vi "BT3562_CMD.vi"(8 "errin":errorcluster caption="entrée d'erreur (pas d'erreur)") -> (0 "errout":errorcluster caption="sortie d'erreur", 3 "Conti (mOhms)":dbl format="%#_10f")   [LabVIEW 2020]
uses:
  <vilib>/Instr/_visa.llb/VISA Find Search Mode.ctl
  <instrlib>/HIOKI BT356X Series/HIOKI BT356X Series.lvlib
panel:
  in  "errin":errorcluster caption="entrée d'erreur (pas d'erreur)"
  in  "visa in":refnum<visa-resource-name>
  out "Conti (Ohms)":dbl format="%#_10f"
  out "VISA OUT":string
  out "DATA OUT":string
  # "DATA OUT"
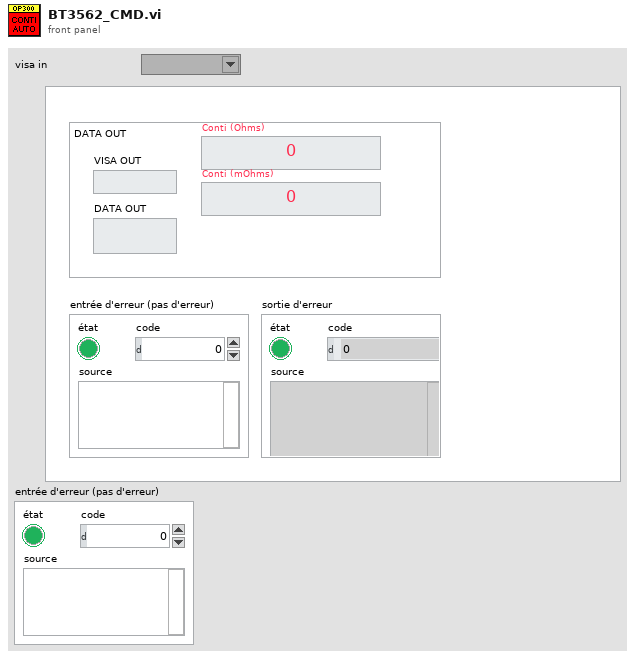
[diagram p1: front panel]
types:
  T1 = typedef "VISA Find Search Mode.ctl" = u32
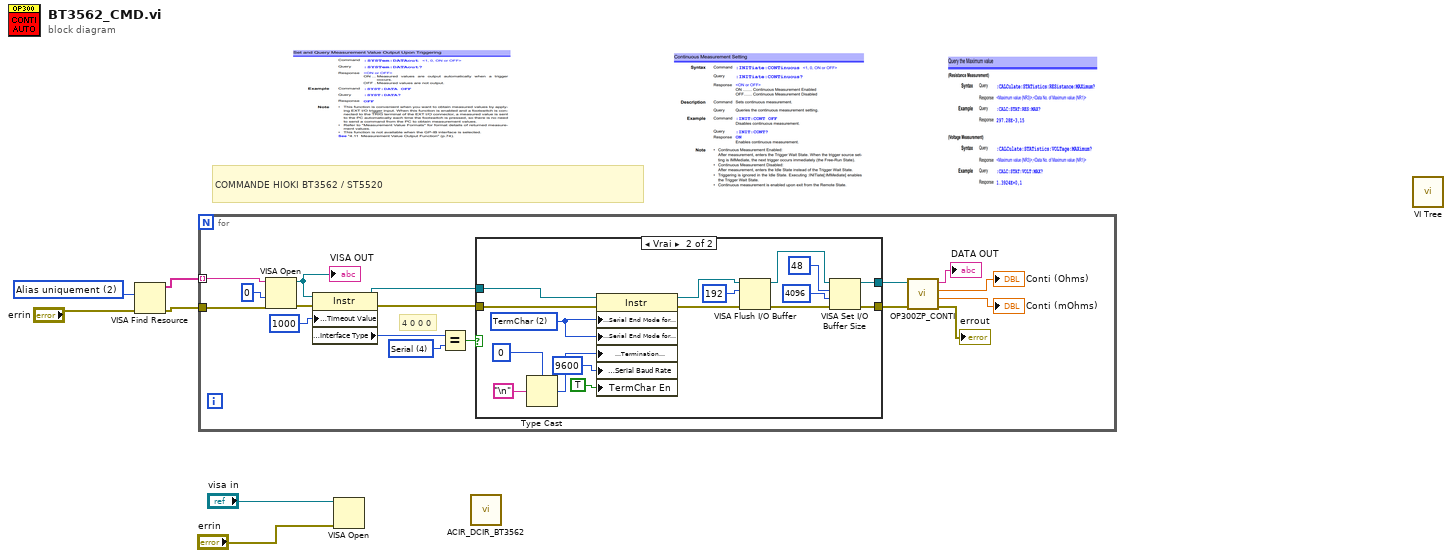
[diagram p0: block diagram]
diagram:
  w6 = T1 2 items=["Noms canoniques uniquement"=0, "Alias uniquement"=2, "Inclure les alias correspondants"=3, "Inclure tous les alias"=4] ("Search Mode")
  # "COMMANDE HIOKI BT3562 / ST5520"
  n1 = VISA Find Resource(8:"errin", 10:w6) -> (0:w4:errorcluster, 3:w5:string[])  [unwired: 1 in, 1 out]
  n2 = for {
    tunnel: w5 -> [w17] mode=indexing
    tunnel: w4 -> [w12]
    w19 = u16 4 items=["GPIB"=1, "VXI"=2, "GPIB-VXI"=3, "Serial"=4, "PXI"=5, "TCPIP"=6, "USB"=7] ("Interface Information:Interface Type")
    # "4 0 0 0"
    n3 = VISA Open(access mode=u32 0, error in (no error)=w12, VISA resource name=w17) -> (VISA resource name=w21:refnum<visa-resource-name>, error out=w20:errorcluster)  [unwired: 2 in]
    "VISA OUT" <- w21
    n4 = property class="Instr"(reference=w21, error in=w20, "General Settings:Timeout Value"=u32 1000) -> (reference out=w15:refnum<visa-resource-name>, error out=w14:errorcluster, "Interface Information:Interface Type"=w18:u16)
    n5 = Equal?(x=w18, y=w19) -> (x = y?=w16:bool)
    n6 = case shown="Vrai" w16 {
      tunnel: [w24 w26] -> w7
      tunnel: [w25 w27] -> w13
      tunnel: w15 -> [w24 w41]
      tunnel: w14 -> [w25 w42]
      frame False {
        # "EDIT: Remove interfaces not supported by your instrument."
        # "GPIB, TCP/IP, and USB Interface"
      }
      frame True {
        w31 = u16 2 items=["None", "LastBit", "TermChar"] ("Serial Settings:Serial End Mode for Reads")
        n7 = Type Cast(type=u8 0, x="\n" ("Line Feed Constant")) -> (*(type *) &x=w30:u8)
        n8 = property class="Instr"(reference=w41, error in=w42, "Serial Settings:Serial End Mode for Reads"=w31, "Serial Settings:Serial End Mode for Writes"=w31, "Message Based Settings:Termination Character"=w30, "Serial Settings:Serial Baud Rate"=u32 9600 ("Serial Settings:Baud Rate"), "TermChar En"=TRUE ("Message Based Settings:Termination Character Enable")) -> (reference out=w37:refnum<visa-resource-name>, error out=w39:errorcluster)
        n9 = VISA Flush I/O Buffer(VISA resource name=w37, mask (16)=u16 192, error in (no error)=w39) -> (VISA resource name out=w40:refnum<visa-resource-name>, error out=w38:errorcluster)
        n10 = VISA Set I/O Buffer Size(VISA resource name=w40, mask (16)=u16 48, size (4096)=u32 4096 ("size (0)"), error in (no error)=w38) -> (VISA resource name out=w26:refnum<visa-resource-name>, error out=w27:errorcluster)
      }
    }
    n11 = call "OP300ZP_CONTI.vi"("VISA"=w7, "ERRIN"=w13) -> ("DATA OUT"=→"DATA OUT":string, "Conti (mOhms)"=→"Conti (Ohms)":dbl, "Conti (Ohms)"=→"Conti (mOhms)":dbl, "ERROUT2"=→"errout":errorcluster)  [unwired: 5 in]
  }
  n12 = VISA Open(error in (no error)="errin", VISA resource name="visa in") -> ()  [unwired: 3 in, 2 out]
  n13 = call <userlib>:"ACIR_DCIR_BT3562.vi"() -> ()  [unwired: 5 in, 7 out]
  n14 = call <instrlib>:"VI Tree.vi"() -> ()  [unwired: 12 in]
